vi "TCP-IP Write-Read.vi"(6 "bytes to read":i32=20, 7 "UDP?":bool, 8 "Error In":errorcluster, 9 "data in":string="*IDN?\r\n", 10 "remote port or service name":u16=5000, 11 "address":string="130.55.69.9") -> (0 "Error Out":errorcluster, 3 "data out":string="Cryo-con,22C,204731,")   [LabVIEW 2015]
panel:
  out "lo(x) 2":u8
  out "hi(x) 2":u8
  out "lo(x)":u8
  out "hi(x)":u8
  in  "milliseconds to wait":u32=100
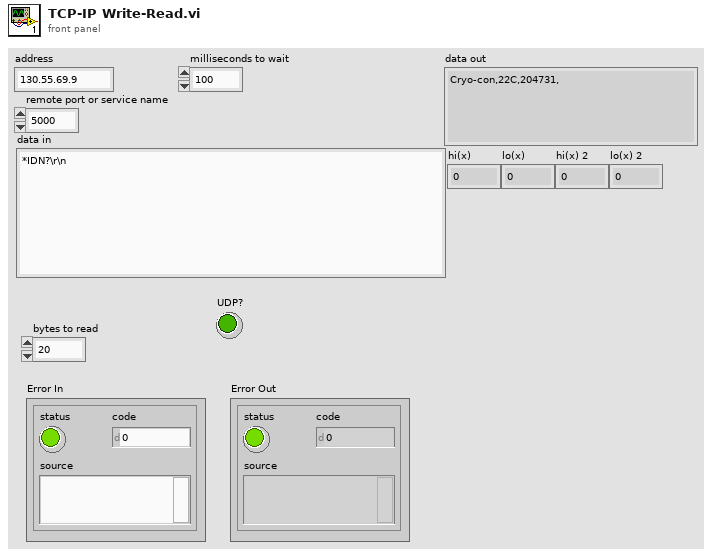
[diagram p1: front panel]
types:
  T1 = enum16{"Standard", "Buffered", "CRLF", "Immediate"}
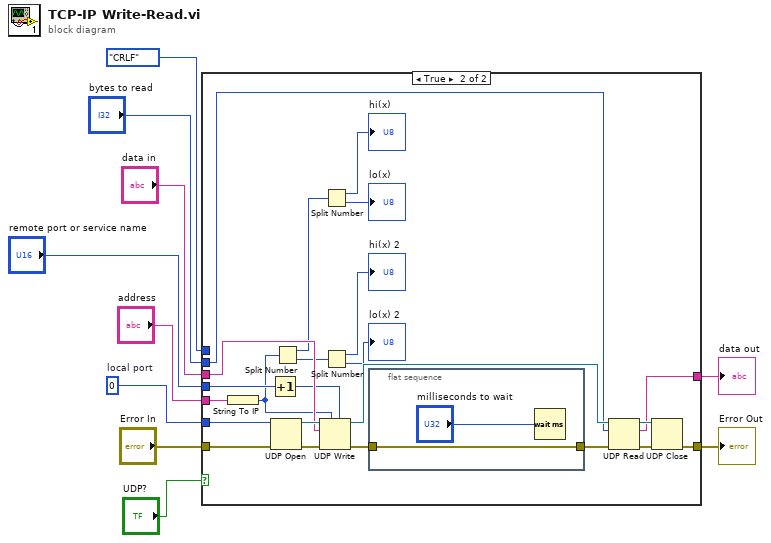
[diagram p0: block diagram]
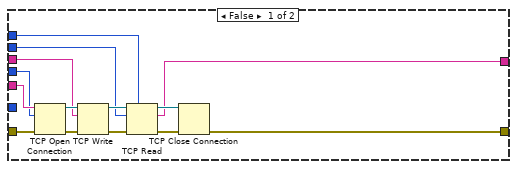
[diagram p2: hidden frame]
diagram:
  w1 = u16 0  # local port
  n1 = case shown="True" "UDP?" {
    tunnel: "address" -> [w24 w38]
    tunnel: "remote port or service name" -> [w17 w35]
    tunnel: "data in" -> [w16 w42]
    tunnel: "bytes to read" -> [w15 w37]
    tunnel: [w14 w41] -> w6
    tunnel: T1."CRLF" ("mode (standard)") -> [w13 _]
    tunnel: [w12 w40] -> w4
    tunnel: "Error In" -> [w11 w39]
    tunnel: w1 -> [_ w36]
    frame False {
      n2 = TCP Open Connection(address=w24, remote port or service name=w17, error in (no error)=w11) -> (connection ID=w23:refnum<k5>, error out=w21:errorcluster)  [unwired: 2 in]
      n3 = TCP Write(connection ID=w23, data in=w16, error in (no error)=w21) -> (connection ID out=w22:refnum<k5>, error out=w20:errorcluster)  [unwired: 1 in, 1 out]
      n4 = TCP Read(connection ID=w22, bytes to read=w15, error in (no error)=w20, 7:w13) -> (connection ID out=w19:refnum<k5>, data out=w14:string, error out=w18:errorcluster)  [unwired: 1 in]
      n5 = TCP Close Connection(connection ID=w19, error in (no error)=w18) -> (error out=w12:errorcluster)  [unwired: 1 in, 1 out]
    }
    frame True {
      n6 = String To IP(1:w38) -> (0:w26:u32)
      n7 = Increment(x=w35) -> (x+1=w25:u16)
      n8 = UDP Open(8:w39, 11:w36) -> (port=w47:refnum<k16>, 0:w45:errorcluster)  [unwired: 3 in, 1 out]
      n9 = Split Number(x=w26) -> (hi(x)=w32:u16, lo(x)=w31:u16)
      n10 = UDP Write(address=w26, port or service name=w25, connection ID=w47, data in=w42, 8:w45) -> (error out=w34:errorcluster, 3:w46:refnum<k16>)  [unwired: 1 in]
      n11 = Split Number(x=w32) -> (hi(x)=→"hi(x)":u8, lo(x)=→"lo(x)":u8)
      n12 = Split Number(x=w31) -> (hi(x)=→"hi(x) 2":u8, lo(x)=→"lo(x) 2":u8)
      n13 = flat-sequence {
        tunnel: w34 -> [w49]
        tunnel: [w49] -> w33
        frame #0 {
          n14 = Wait (ms)(milliseconds to wait="milliseconds to wait") -> ()  [unwired: 1 out]
        }
      }
      n15 = UDP Read(connection ID=w46, max size (548)=w37, 8:w33) -> (data out=w41:string, error out=w43:errorcluster, 3:w44:refnum<k16>)  [unwired: 1 in, 2 out]
      n16 = UDP Close(connection ID=w44, 8:w43) -> (error out=w40:errorcluster)  [unwired: 1 out]
    }
  }
  "data out" <- w6
  "Error Out" <- w4
